vi "RT_Release.vi"(8 "error in":errorcluster, 11 "Main Data":T1) -> (0 "error out":errorcluster)   [LabVIEW 2018]
uses:
  Data Def/RT_Main Data.ctl
  Data Def/RT_FPGA VI Reference.ctl
  Data Def/RT_Request Data.ctl
  <vilib>/FPGAPlugInAG/Dynamic/niLvFpga_Close_Dynamic.vi
  <vilib>/rvi/interface/nirviCloseFPGA/nirviCloseFPGA.xnode
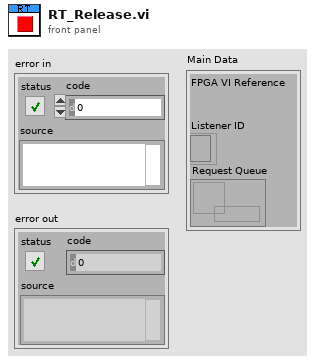
[diagram p1: front panel]
types:
  T1 = typedef "RT_Main Data.ctl" = cluster{"FPGA VI Reference":T2, "Listener ID":refnum<k5>, "Request Queue":refnum<queue>}
  T2 = typedef "RT_FPGA VI Reference.ctl" = refnum<k20>
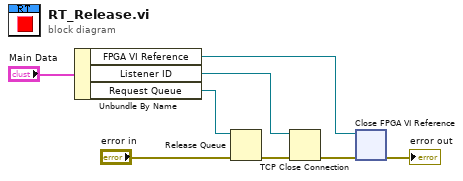
[diagram p0: block diagram]
diagram:
  n1 = Unbundle By Name("Main Data") -> ("FPGA VI Reference"=w3:T2, "Listener ID"=w5:refnum<k5>, "Request Queue"=w7:refnum<queue>)
  n2 = Release Queue(queue=w7, error in (no error)="error in") -> (error out=w6:errorcluster)  [unwired: 1 in, 2 out]
  n3 = TCP Close Connection(connection ID=w5, error in (no error)=w6) -> (error out=w4:errorcluster)  [unwired: 1 in, 1 out]
  n4 = xnode "Close FPGA VI Reference"("FPGA VI Reference In"=w3, "error in"=w4) -> ("error out"=→"error out":errorcluster)
